vi "Construct_Extract_pair_testing.vi"() -> ()   [LabVIEW 2019, in "mmW_commands.lvlib"]
uses:
  mmW_commands.lvlib
panel:
  out "error out":errorcluster
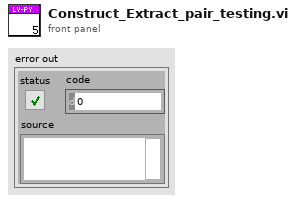
[diagram p1: front panel]
types:
  T1 = typedef "mmW_commands.lvlib/command_types.ctl" = enum16{"invalid_command", "instrument_control", "environment_control", "response"}
  T2 = typedef "mmW_commands.lvlib/commands.ctl" = enum16{"configure_fs", "configure_rf", "configure_trigger", "equalization_enable", "equalization_start", "lo_sync_enable", "equalization_stop", "get_instrument_status", "get_versions", "initialize_hw", "pop_rx", "set_log_level", "Shutdown", "start", "start_instrument_app", "stop", "trans", "transceive", "trigger_burst", "trigger_sync_enable", "Write TX", "resp_generic", "resp_waveform", "send_trigger", "fetch", "transceive2"}
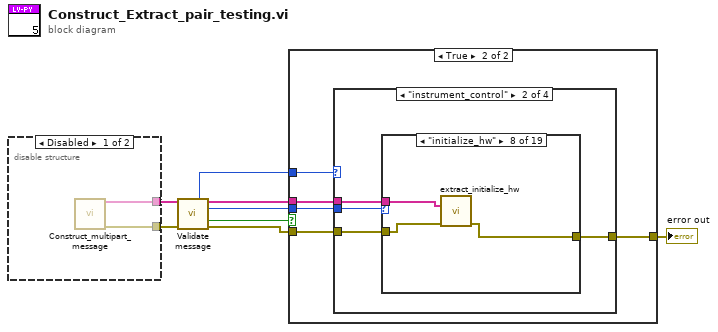
[diagram p0: block diagram]
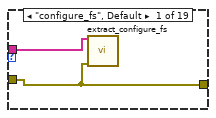
[diagram p5: hidden frame]
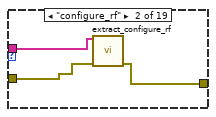
[diagram p6: hidden frame]
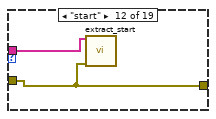
[diagram p15: hidden frame]
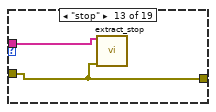
[diagram p16: hidden frame]
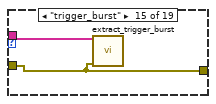
[diagram p18: hidden frame]
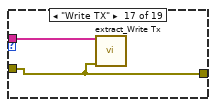
[diagram p20: hidden frame]
diagram:
  n1 = disable-structure shown="Disabled" {
    disable-tunnel: [w10 _] -> w8
    disable-tunnel: [w9 _] -> w5
    frame Disabled {
      n2 = call "Construct_multipart_message.vi"() -> ("Multipart message"=w10:string[], "error out"=w9:errorcluster)  [unwired: 12 in, 2 out]
    }
    frame Enabled {
    }
  }
  n3 = call "Validate message.vi"("multipart message in"=w8, "error in (no error)"=w5) -> ("Command Type"=w2:T1, "multipart message out"=w7:string[], "command out"=w3:T2, "Valid message?"=w6:bool, "error out"=w4:errorcluster)  [unwired: 8 in, 1 out]
  n4 = case shown="True" w6 {
    tunnel: w7 -> [_ w16]
    tunnel: w4 -> [w11 w15]
    tunnel: [w11 w14] -> w1
    tunnel: w3 -> [_ w13]
    tunnel: w2 -> [_ w12]
    frame False {
    }
    frame True {
      n5 = case shown="\"instrument_control\"" w12 {
        tunnel: w16 -> [_ w21 _ _]
        tunnel: w15 -> [w17 w20 w50 w51]
        tunnel: [w17 w19 w50 w51] -> w14
        tunnel: w13 -> [_ w18 _ _]
        frame "invalid_command", Default {
        }
        frame "instrument_control" {
          n6 = case shown="\"initialize_hw\"" w18 {
            tunnel: w21 -> [w23 w26 _ _ _ _ _ w32 _ _ _ w39 w41 _ w44 _ w46 _ _]
            tunnel: w20 -> [w22 w25 w27 w28 w29 w30 w31 w34 w35 w36 w37 w38 w40 w42 w43 w45 w47 w48 w49]
            tunnel: [w22 w24 w27 w28 w29 w30 w31 w33 w35 w36 w37 w38 w40 w42 w43 w45 w47 w48 w49] -> w19
            frame "configure_fs", Default {
              n7 = call "extract_configure_fs.vi"("multipart message in"=w23, "error in (no error)"=w22) -> ()  [unwired: 9 in, 5 out]
            }
            frame "configure_rf" {
              n8 = call "extract_configure_rf.vi"("multipart message in"=w26, "error in (no error)"=w25) -> ("error out"=w24:errorcluster)  [unwired: 8 in, 5 out]
            }
            frame "configure_trigger" {
            }
            frame "equalization_enable" {
            }
            frame "equalization_start" {
            }
            frame "lo_sync_enable" {
            }
            frame "equalization_stop" {
            }
            frame "initialize_hw" {
              n9 = call "extract_initialize_hw.vi"("multipart message in"=w32, "error in (no error)"=w34) -> ("error out"=w33:errorcluster)  [unwired: 9 in, 4 out]
            }
            frame "pop_rx" {
            }
            frame "set_log_level" {
            }
            frame "Shutdown" {
            }
            frame "start" {
              n10 = call "extract_start.vi"("multipart message in"=w39, "error in (no error)"=w38) -> ()  [unwired: 9 in, 5 out]
            }
            frame "stop" {
              n11 = call "extract_stop.vi"("multipart message in"=w41, "error in (no error)"=w40) -> ()  [unwired: 11 in, 3 out]
            }
            frame "transceive" {
            }
            frame "trigger_burst" {
              n12 = call "extract_trigger_burst.vi"("multipart message in"=w44, "error in (no error)"=w43) -> ()  [unwired: 9 in, 5 out]
            }
            frame "trigger_sync_enable" {
            }
            frame "Write TX" {
              n13 = call "extract_Write Tx.vi"("multipart message in"=w46, "error in (no error)"=w47) -> ()  [unwired: 8 in, 6 out]
            }
            frame "resp_generic" {
            }
            frame "resp_waveform" {
            }
          }
        }
        frame "environment_control" {
        }
        frame "response" {
        }
      }
    }
  }
  "error out" <- w1
